vi "Common-AbsLessThan.vi"(9 "u":dbl, 10 "y":dbl, 11 "x":dbl) -> (3 "abs(x-y) < u?":bool)   [LabVIEW 2014]
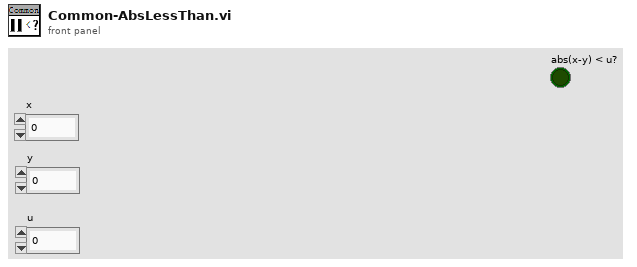
[diagram p1: front panel]
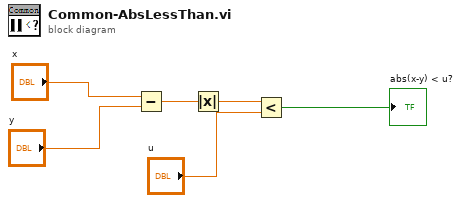
[diagram p0: block diagram]
diagram:
  n1 = Subtract(x="x", y="y") -> (x-y=w6:dbl)
  n2 = Absolute Value(x=w6) -> (abs(x)=w5:dbl)
  n3 = Less?(x=w5, y="u") -> (x < y?=→"abs(x-y) < u?":bool)
